vi "test_unwrap_phase.vi"() -> ()   [LabVIEW 2013]
uses:
  <vilib>/Analysis/NI_AALPro.lvlib
panel:
  out "size(s)":i32[](array[numeric])
  out "Waveform Chart":dbl[][](graph)
  out "Phase":dbl[][](array[numeric])
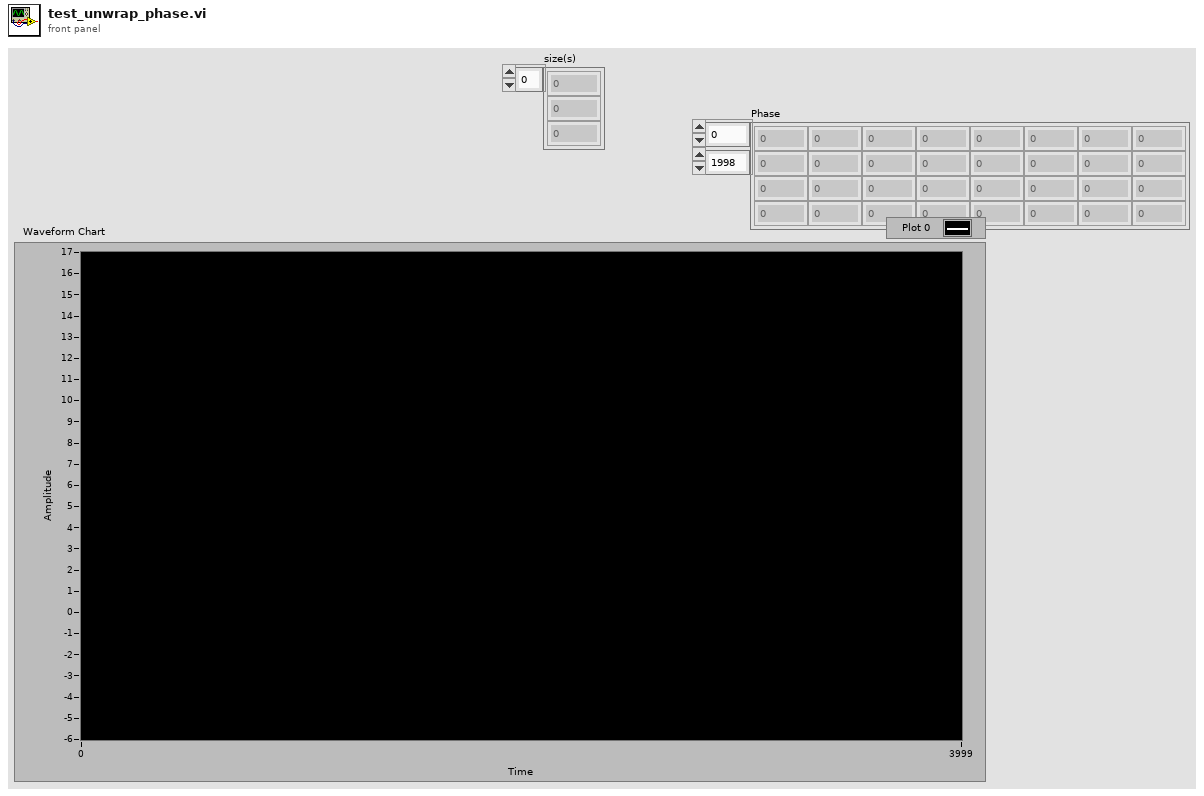
[diagram p1: front panel]
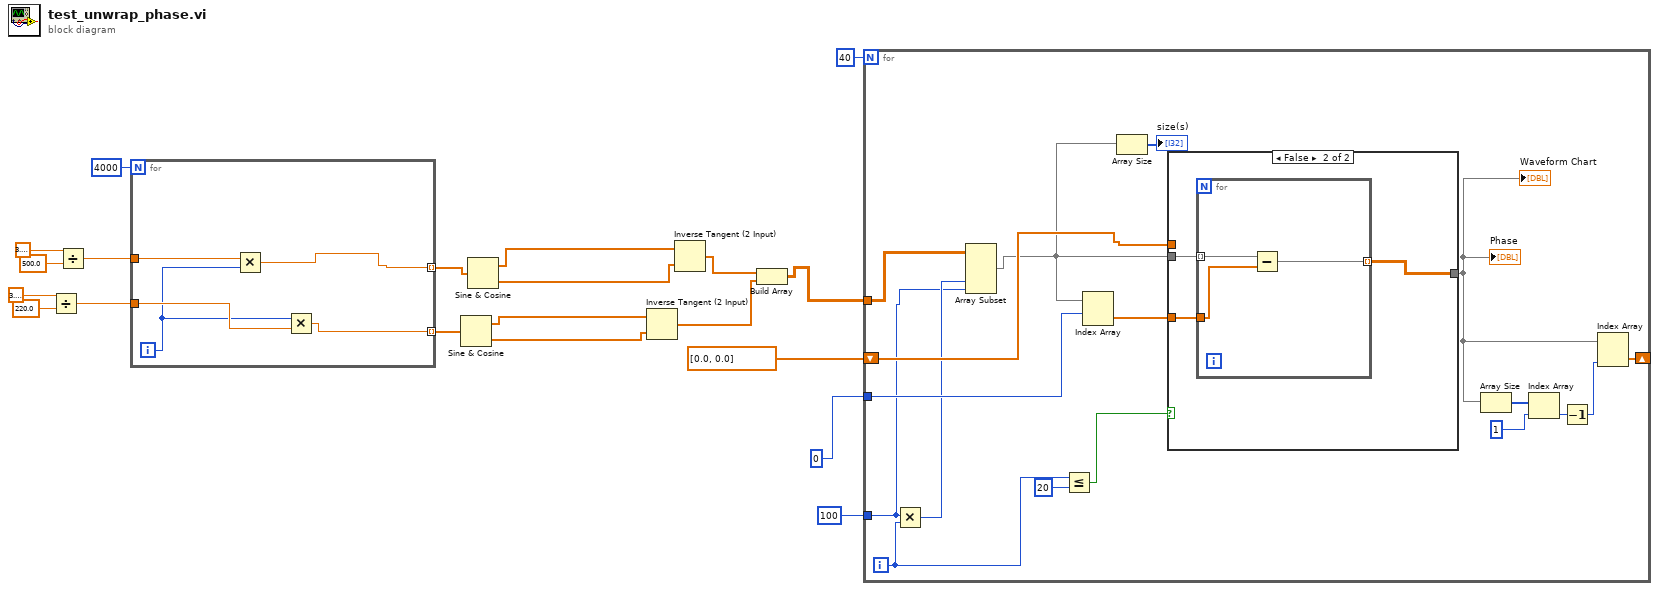
[diagram p0: block diagram]
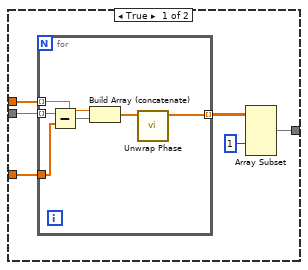
[diagram p2: hidden frame]
diagram:
  n1 = Divide(x=3.141592653589793, y=220.0) -> (x/y=w11:dbl)
  n2 = Divide(x=3.141592653589793, y=500.0) -> (x/y=w16:dbl)
  n3 = for {
    N: 4000 -> [_]
    tunnel: [w24] -> w17 mode=indexing
    tunnel: w16 -> [w25]
    tunnel: w11 -> [w23]
    tunnel: [w21] -> w10 mode=indexing
    i -> [w22]
    n4 = Multiply(x=w25, y=w22) -> (x*y=w24:dbl)
    n5 = Multiply(x=w22, y=w23) -> (x*y=w21:dbl)
  }
  n6 = Sine & Cosine(0:w10) -> (1:w9:dbl[], 2:w8:dbl[])
  n7 = Sine & Cosine(0:w17) -> (1:w15:dbl[], 2:w14:dbl[])
  n8 = Inverse Tangent (2 Input)(1:w8, 2:w9) -> (0:w6:dbl[])
  n9 = Inverse Tangent (2 Input)(1:w14, 2:w15) -> (0:w7:dbl[])
  n10 = Build Array(w7, w6) -> (w5:dbl[][])
  n11 = for {
    N: 40 -> [_]
    shift-right: [w39] -> _
    shift-left: dbl[] [0.0, 0.0] -> [w36]
    tunnel: 0 -> [w35]
    tunnel: w5 -> [w33]
    tunnel: 100 -> [w30]
    i -> [w28]
    n12 = Multiply(x=w30, y=w28) -> (x*y=w31:i32)
    n13 = Array Subset(array=w33, index (col)=w31, length (col)=w30) -> (w29:dbl[][])  [unwired: 2 in]
    n14 = Less Or Equal?(x=w28, y=20) -> (x <= y?=w26:bool)
    n15 = Index Array(array=w29, index (row)=w35) -> (element=w42:dbl[])  [unwired: 1 in]
    n16 = Array Size(array=w29) -> (size(s)=→"size(s)":i32[])
    n17 = case shown="False" w26 {
      tunnel: w42 -> [w48 w57]
      tunnel: w36 -> [w47 _]
      tunnel: [w44 w55] -> w34
      tunnel: w29 -> [w43 w56]
      frame True {
        n18 = for {
          tunnel: w43 -> [w54] mode=indexing
          tunnel: w48 -> [w53]
          tunnel: [w52] -> w45 mode=indexing
          tunnel: w47 -> [w50] mode=indexing
          n19 = Subtract(x=w54, y=w53) -> (x-y=w51:dbl[])
          n20 = Build Array (concatenate)(w50, w51) -> (w49:dbl[])
          n21 = call <vilib>:"Unwrap Phase.vi"("Phase"=w49) -> ("Unwrapped Phase"=w52:dbl[])  [unwired: 9 in, 1 out]
        }
        n22 = Array Subset(array=w45, index (col)=1 ("index")) -> (w44:dbl[][])  [unwired: 3 in]
      }
      frame False {
        n23 = for {
          tunnel: w56 -> [w60] mode=indexing
          tunnel: w57 -> [w59]
          tunnel: [w58] -> w55 mode=indexing
          n24 = Subtract(x=w60, y=w59) -> (x-y=w58:dbl[])
        }
      }
    }
    "Phase" <- w34
    "Waveform Chart" <- w34
    n25 = Array Size(array=w34) -> (size(s)=w41:i32[])
    n26 = Index Array(array=w41, index=1) -> (element=w40:i32)
    n27 = Decrement(x=w40) -> (x-1=w38:i32)
    n28 = Index Array(array=w34, index (col)=w38) -> (element=w39:dbl[])  [unwired: 1 in]
  }
